vi "_PC_RTLoop_Save_Log_Data.vi"(8 "error in (no error)":errorcluster, 10 "data array of string":string[](array[string])) -> (0 "error out":errorcluster)   [LabVIEW 2018]
uses:
  Constant/AccessFolderName.ctl
  <vilib>/Utility/file.llb/Read Delimited Spreadsheet (string).vi
  <vilib>/Utility/file.llb/Write Delimited Spreadsheet (string).vi
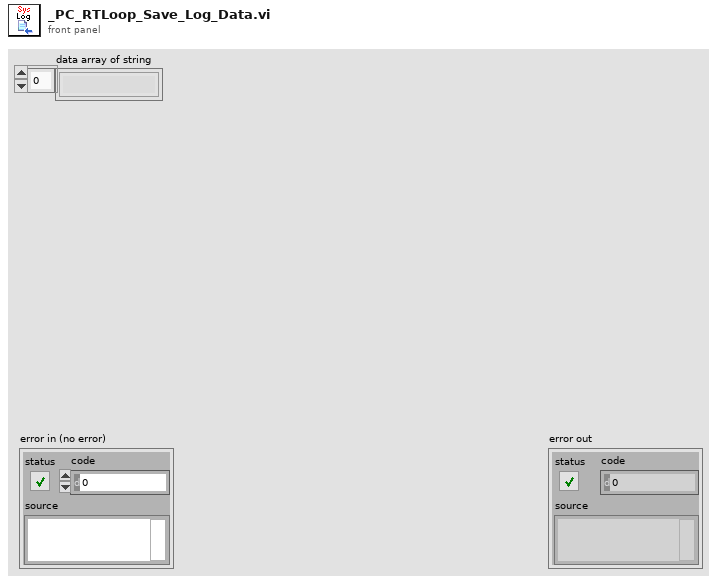
[diagram p1: front panel]
types:
  T1 = typedef "AccessFolderName.ctl" = enum16{"None", "system_log", "ui_log", "msdata", "method", "d999_param"}
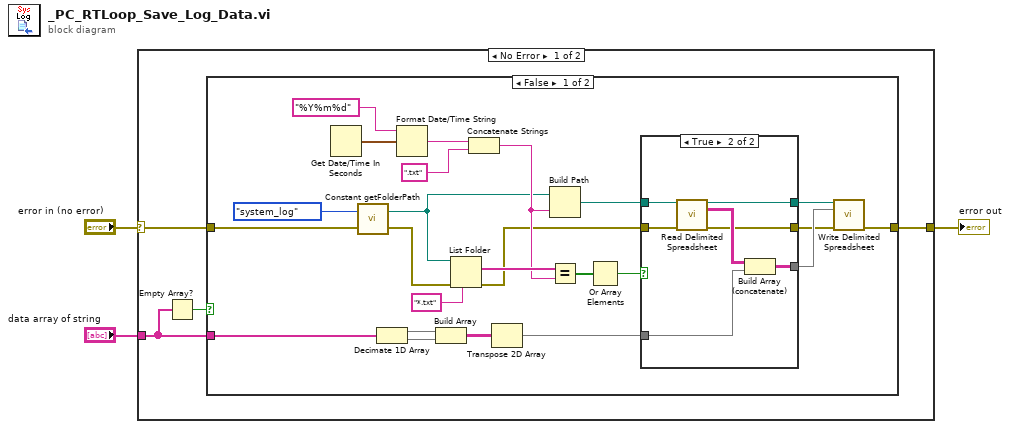
[diagram p0: block diagram]
diagram:
  n1 = case shown="No Error" "error in (no error)" {
    selector: "error in (no error)" -> [w4 w43]
    tunnel: [w7 w43] -> w3
    tunnel: "data array of string" -> [w6 _]
    frame No Error {
      n2 = Empty Array?(array=w6) -> (empty?=w5:bool)
      n3 = case shown="False" w5 {
        tunnel: [w10 w42] -> w7
        tunnel: w6 -> [w9 _]
        tunnel: w4 -> [w8 w42]
        frame False {
          n4 = Get Date/Time In Seconds() -> (seconds since 1Jan1904=w30:timestamp)
          n5 = call "Constant getFolderPath.vi"("error in (no error)"=w8, "folder name"=AccessFolderName."system_log") -> ("error out"=w11:errorcluster, "folder path"=w12:path)
          n6 = Decimate 1D Array(w9) -> (w17:string[], w16:string[])
          n7 = Format Date/Time String(time format string (%c)="%Y%m%d", seconds (now)=w30) -> (date/time string=w27:string)  [unwired: 1 in]
          n8 = Build Array(w17, w16) -> (w15:string[][])
          n9 = List Folder(path=w12, pattern="*.txt", error in=w11) -> (filenames=w28:string[], error out=w18:errorcluster)  [unwired: 1 in, 2 out]
          n10 = Concatenate Strings(w27, ".txt" ("name or relative path")) -> (w23:string)
          n11 = Transpose 2D Array(2D array=w15) -> (transposed array=w14:string[][])
          n12 = Build Path(base path=w12, name or relative path=w23) -> (appended path=w22:path)
          n13 = Equal?(x=w28, y=w23) -> (x = y?=w25:bool[])
          n14 = Or Array Elements(Boolean array=w25) -> (logical OR=w24:bool)
          n15 = case shown="True" w24 {
            tunnel: w22 -> [w33 w41]
            tunnel: w14 -> [w34 w39]
            tunnel: [w34 w38] -> w20
            tunnel: [w33 w37] -> w21
            tunnel: [w32 w36] -> w19
            tunnel: w18 -> [w32 w35]
            frame False {
            }
            frame True {
              n16 = call-poly <vilib>:"Read Delimited Spreadsheet.vi"("file path (dialog if empty)"=w41, "error in (no error)"=w35) -> ("new file path (Not A Path if cancelled)"=w37:path, "all rows"=w40:string[][], "error out"=w36:errorcluster)  [unwired: 8 in, 3 out]
              n17 = Build Array (concatenate)(w40, w39) -> (w38:string[][])
            }
          }
          n18 = call-poly <vilib>:"Write Delimited Spreadsheet.vi"("file path (dialog if empty)"=w21, "2D data"=w20, "error in (no error)"=w19) -> ("error out"=w10:errorcluster)  [unwired: 11 in, 1 out]
        }
        frame True {
        }
      }
    }
    frame Error {
    }
  }
  "error out" <- w3
